vi "T_B_write.vi"(6 "refnum":refnum<file>) -> ()   [LabVIEW 2016]
uses:
  Instrument_Setup.vi
  Global Variables/Data_Display_global.vi
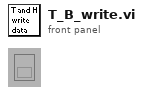
[diagram p1: front panel]
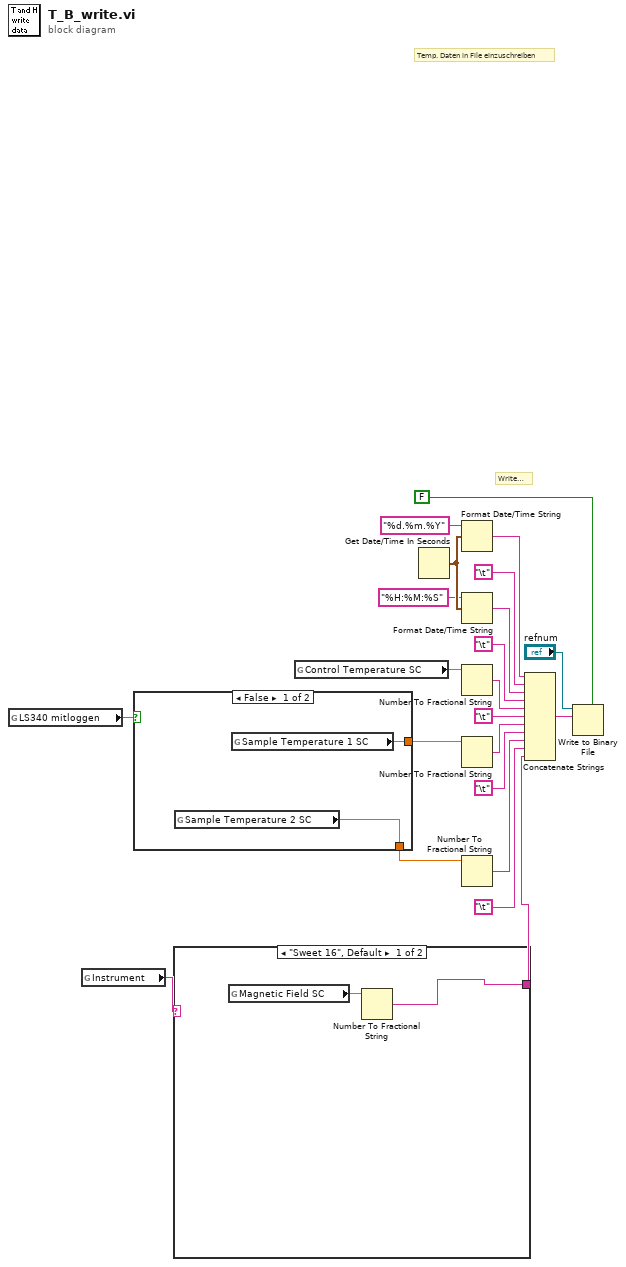
[diagram p0: block diagram]
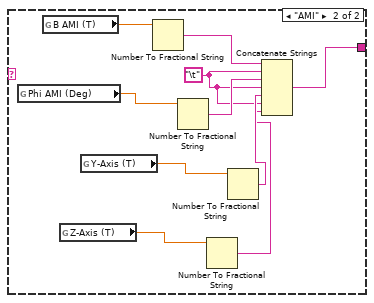
[diagram p2: hidden frame]
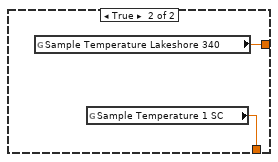
[diagram p3: hidden frame]
diagram:
  # "Temp. Daten in File einzuschreiben"
  # "Write File"
  n1 = global read "Instrument_Setup.vi" "LS340 mitloggen"() -> (w14)
  n2 = global read "Instrument_Setup.vi" "Instrument"() -> (w1:string)
  n3 = case shown="False" w14 {
    tunnel: [w24 w26] -> w15
    tunnel: [w23 w25] -> w4
    frame False {
      n4 = global read "Data_Display_global.vi" "Sample Temperature 2 SC"() -> (w23:dbl)
      n5 = global read "Data_Display_global.vi" "Sample Temperature 1 SC"() -> (w24:dbl)
    }
    frame True {
      n6 = global read "Data_Display_global.vi" "Sample Temperature Lakeshore 340"() -> (w26:dbl)
      n7 = global read "Data_Display_global.vi" "Sample Temperature 1 SC"() -> (w25:dbl)
    }
  }
  n8 = case shown="\"Sweet 16\", Default" w1 {
    tunnel: [w27 w34] -> w2
    frame "Sweet 16", Default {
      n9 = global read "Data_Display_global.vi" "Magnetic Field SC"() -> (w28:dbl)
      n10 = Number To Fractional String(number=w28) -> (F-format string=w27:string)  [unwired: 3 in]
    }
    frame "AMI" {
      w29 = "\t"
      n11 = global read "Data_Display_global.vi" "Phi AMI (Deg)"() -> (w37:dbl)
      n12 = global read "Data_Display_global.vi" "B AMI (T)"() -> (w38:dbl)
      n13 = global read "Data_Display_global.vi" "Z-Axis (T)"() -> (w32:dbl)
      n14 = global read "Data_Display_global.vi" "Y-Axis (T)"() -> (w33:dbl)
      n15 = Number To Fractional String(number=w38) -> (F-format string=w36:string)  [unwired: 3 in]
      n16 = Number To Fractional String(number=w37) -> (F-format string=w35:string)  [unwired: 3 in]
      n17 = Number To Fractional String(number=w32) -> (F-format string=w30:string)  [unwired: 3 in]
      n18 = Number To Fractional String(number=w33) -> (F-format string=w31:string)  [unwired: 3 in]
      n19 = Concatenate Strings(w36, w29, w35, w29, w31, w29, w30) -> (w34:string)
    }
  }
  n20 = global read "Data_Display_global.vi" "Control Temperature SC"() -> (w10:dbl)
  n21 = Get Date/Time In Seconds() -> (seconds since 1Jan1904=w8:timestamp)
  n22 = Format Date/Time String(time format string (%c)="%d.%m.%Y", seconds (now)=w8) -> (date/time string=w6:string)  [unwired: 1 in]
  n23 = Format Date/Time String(time format string (%c)="%H:%M:%S", seconds (now)=w8) -> (date/time string=w5:string)  [unwired: 1 in]
  n24 = Number To Fractional String(number=w10) -> (F-format string=w17:string)  [unwired: 3 in]
  n25 = Number To Fractional String(number=w15) -> (F-format string=w18:string)  [unwired: 3 in]
  n26 = Number To Fractional String(number=w4) -> (F-format string=w19:string)  [unwired: 3 in]
  n27 = Concatenate Strings(w6, "\t", w5, "\t", w17, "\t", w18, "\t", w19, "\t", w2) -> (w13:string)
  n28 = Write to Binary File(file (use dialog)="refnum", data=w13, 5:FALSE ("prepend array or string size? (T)")) -> ()  [unwired: 3 in, 3 out]
